vi "Get cyclic instructions.vi"(8 "error in (no error)":errorcluster, 10 "cyclic parameter":string, 11 "Motor in":refnum<class "Motor.lvclass">) -> (0 "error out":errorcluster, 1 "start":bool, 2 "cyclic instructions":string[](array[string]), 3 "Motor out":refnum<class "Motor.lvclass">)   [LabVIEW 2018, in "Motor.lvclass"]
uses:
  Motor.lvclass
  Motor.lvclass/Motor.ctl
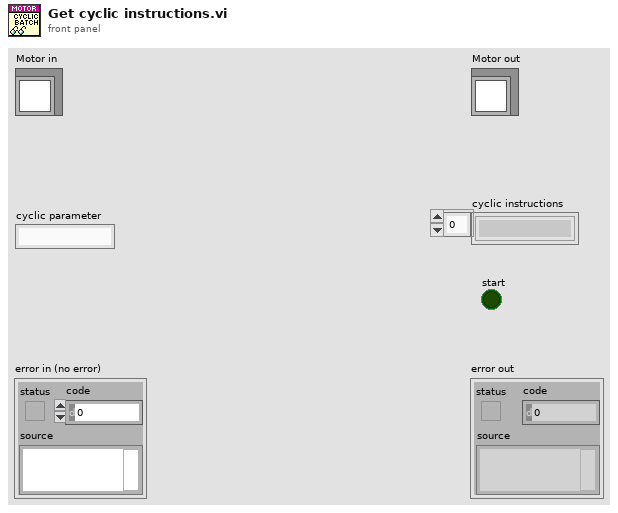
[diagram p1: front panel]
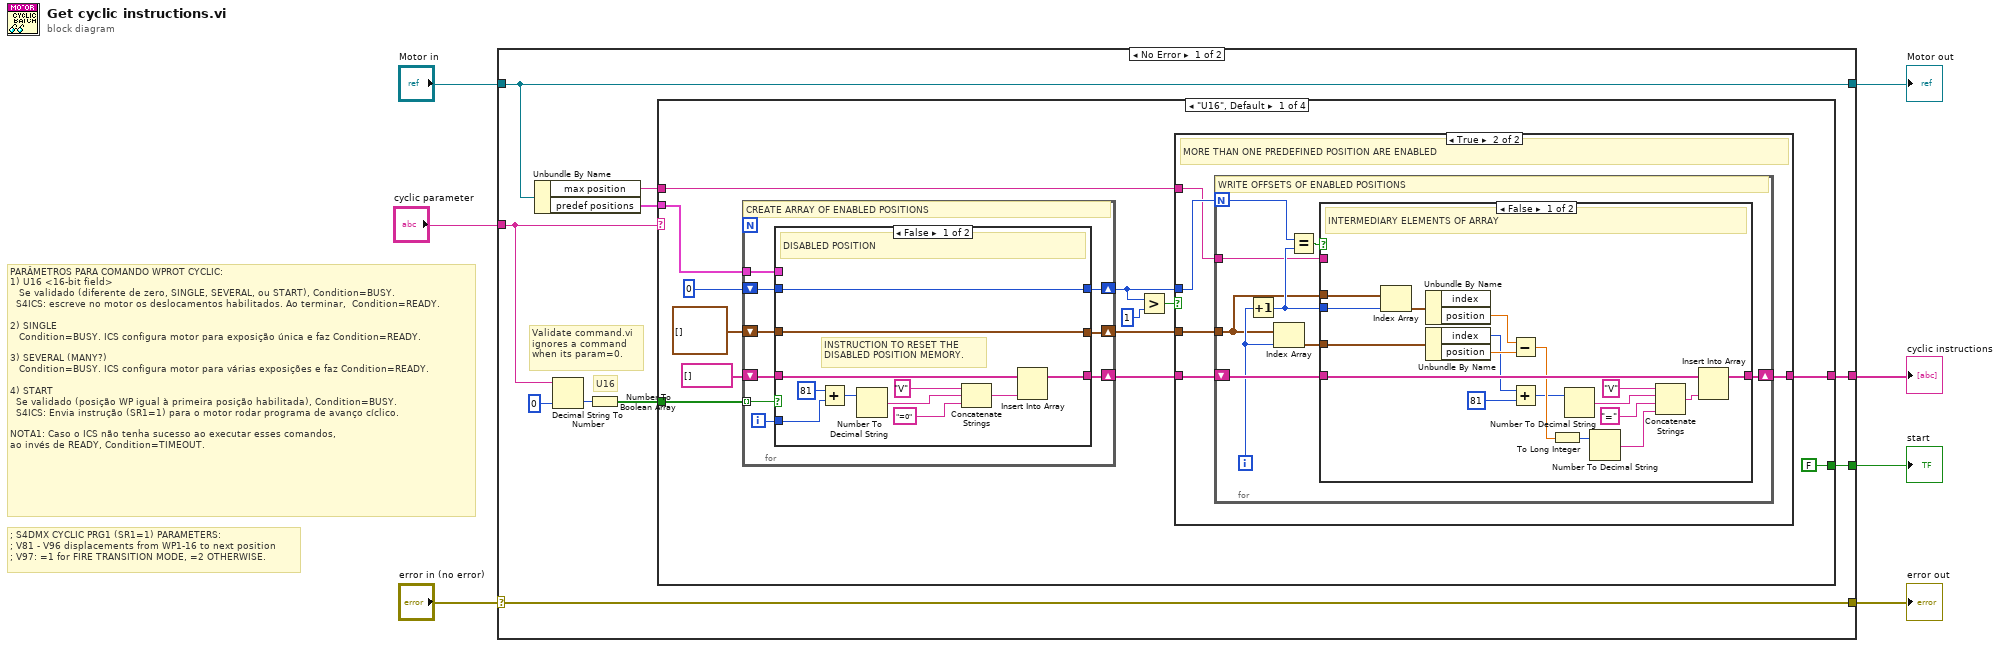
[diagram p0: block diagram]
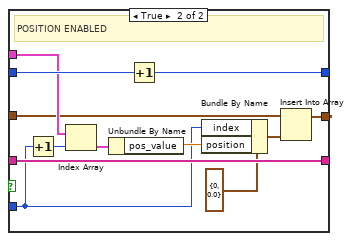
[diagram p2: hidden frame]
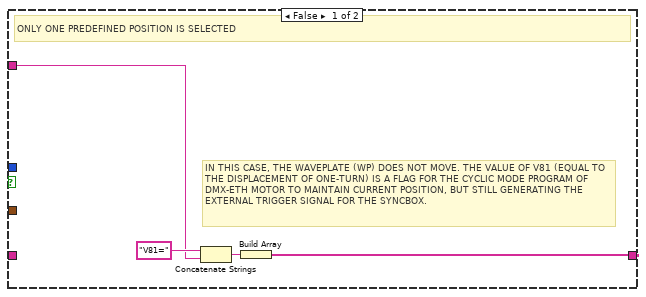
[diagram p3: hidden frame]
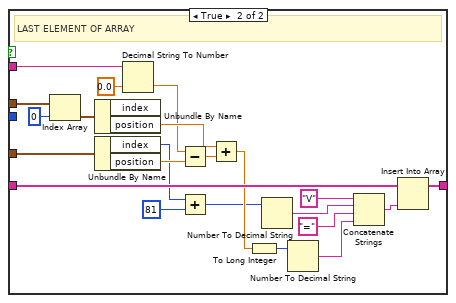
[diagram p4: hidden frame]
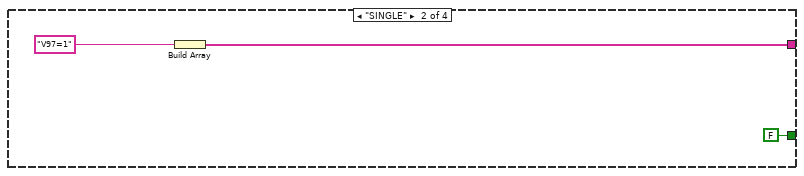
[diagram p5: hidden frame]
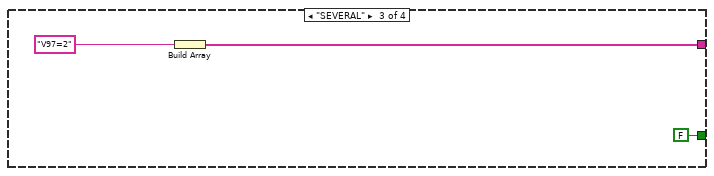
[diagram p6: hidden frame]
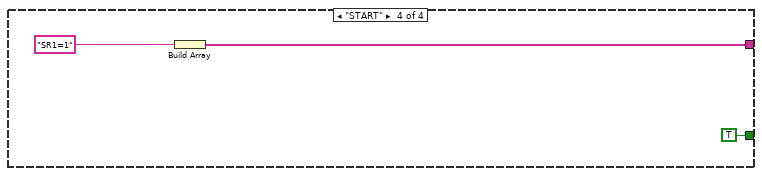
[diagram p7: hidden frame]
diagram:
  # "; S4DMX CYCLIC PRG1 (SR1=1) PARAMETERS:\n; V81 - V96 displacements from WP1-16 to next position\n; V97: =1 for FIRE TRANSITION MODE, =2 OTHERWISE."
  # "PARÂMETROS PARA COMANDO WPROT CYCLIC:\n1) U16 <16-bit field>\n   Se validado (diferente de zero, SINGLE, SEVERAL, ou START), Condition=BUSY.\n  S4ICS: escreve no motor os deslocamentos habilitados. Ao terminar,  Condition=READY.\n\n2) SINGLE\n   Condition=BUSY. ICS configura motor para exposição única e faz Condition=READY.\n\n3) SEVERAL (MANY?)\n   Condition=BUSY. ICS configura motor para várias exposições e faz Condition=READY.\n\n4) START\n  Se validado (posição WP igual à primeira posição habilitada), Condition=BUSY.\n  S4ICS: Envia instrução (SR1=1) para o motor rodar programa de avanço cíclico.\n\nNOTA1: Caso o ICS não tenha sucesso ao executar esses comandos, \nao invés de READY, Condition=TIMEOUT."
  n1 = case shown="No Error" "error in (no error)" {
    selector: "error in (no error)" -> [w17 w130]
    tunnel: [w17 w130] -> w6
    tunnel: [w16 w131] -> w4
    tunnel: "Motor in" -> [w16 w131]
    tunnel: "cyclic parameter" -> [w13 _]
    tunnel: [w9 _] -> w2
    tunnel: [w8 _] -> w1
    frame No Error {
      # "Validate command.vi\nignores a command\nwhen its param=0."
      # "U16"
      n2 = Unbundle By Name(w16) -> ("max position"=w14:string, "predef positions"=w15:cluster{"pos_name":string, "pos_value":dbl}[])
      n3 = Decimal String To Number(string=w13, default (0L)=u16 0) -> (number=w12:u16)  [unwired: 1 in, 1 out]
      n4 = Number To Boolean Array(number=w12) -> (Boolean array=w10:bool[])
      n5 = case shown="\"U16\", Default" w13 {
        tunnel: w15 -> [w26 _ _ _]
        tunnel: w14 -> [w20 _ _ _]
        tunnel: w10 -> [w28 _ _ _]
        tunnel: [w19 w122 w125 w128] -> w9
        tunnel: [FALSE FALSE FALSE TRUE] -> w8
        frame "U16", Default {
          n6 = for {
            tunnel: w28 -> [w37] mode=indexing
            shift-right: [w39] -> w21
            shift-left: u16 0 -> [w38]
            shift-right: [w35] -> w22
            shift-left: string[] [] ("appended array") -> [w36]
            tunnel: w26 -> [w33]
            shift-right: [w31] -> w23
            shift-left: cluster{"index":u16, "position":dbl}[] [] ("enabled array") -> [w32]
            i -> [w34]
            # "CREATE ARRAY OF ENABLED POSITIONS"
            n7 = case shown="False" w37 {
              tunnel: [w50 w62] -> w39
              tunnel: w38 -> [w50 w61]
              tunnel: w36 -> [w43 w60]
              tunnel: [w42 w60] -> w35
              tunnel: w34 -> [w44 w51]
              tunnel: w33 -> [_ w59]
              tunnel: w32 -> [w40 w56]
              tunnel: [w40 w57] -> w31
              frame False {
                # "INSTRUCTION TO RESET THE \nDISABLED POSITION MEMORY."
                # "DISABLED POSITION"
                n8 = Add(x=81, y=w44) -> (x+y=w49:i32)
                n9 = Number To Decimal String(number=w49) -> (decimal integer string=w48:string)  [unwired: 1 in]
                n10 = Concatenate Strings("V", w48, "=0") -> (w41:string)
                n11 = Insert Into Array(array=w43, new element=w41) -> (w42:string[])  [unwired: 1 in]
              }
              frame True {
                # "POSITION ENABLED"
                n12 = Increment(x=w51) -> (x+1=w53:i32)
                n13 = Index Array(array=w59, index=w53) -> (element=w58:cluster{"pos_name":string, "pos_value":dbl})
                n14 = Unbundle By Name(w58) -> ("pos_value"=w54:dbl)
                n15 = Increment(x=w61) -> (x+1=w62:u16)
                n16 = Bundle By Name(cluster=cluster{"index":u16, "position":dbl} {"index"=0, "position"=0.0} ("element"), "index"=w51, "position"=w54) -> (w52:cluster{"index":u16, "position":dbl})
                n17 = Insert Into Array(array=w56, new element=w52) -> (w57:cluster{"index":u16, "position":dbl}[])  [unwired: 1 in]
              }
            }
          }
          n18 = Greater?(x=w21, y=u16 1) -> (0:w30:bool)
          n19 = case shown="True" w30 {
            tunnel: w20 -> [w64 w68]
            tunnel: w23 -> [_ w70]
            tunnel: w22 -> [_ w71]
            tunnel: w21 -> [_ w69]
            tunnel: [w63 w67] -> w19
            frame False {
              # "IN THIS CASE, THE WAVEPLATE (WP) DOES NOT MOVE. THE VALUE OF V81 (EQUAL TO THE DISPLACEMENT OF ONE-TURN) IS A FLAG FOR THE CYCLIC MODE PROGRAM OF DMX-ETH MOTOR TO MAINTAIN CURRENT POSITION, BUT STILL GENERATING THE EXTERNAL TRIGGER SIGNAL FOR THE SYNCBOX."
              # "ONLY ONE PREDEFINED POSITION IS SELECTED"
              n20 = Concatenate Strings("V81=", w64) -> (w66:string)
              n21 = Build Array(w66) -> (w63:string[])
            }
            frame True {
              # "MORE THAN ONE PREDEFINED POSITION ARE ENABLED"
              n22 = for {
                N: w69 -> [w76]
                tunnel: w70 -> [w74]
                shift-right: [w77] -> w67
                shift-left: w71 -> [w79]
                tunnel: w68 -> [w72]
                i -> [w78]
                # "WRITE OFFSETS OF ENABLED POSITIONS"
                n23 = Increment(x=w78) -> (x+1=w75:i32)
                n24 = Index Array(array=w74, index=w78) -> (element=w80:cluster{"index":u16, "position":dbl})
                n25 = Equal?(x=w76, y=w75) -> (x = y?=w73:bool)
                n26 = case shown="False" w73 {
                  tunnel: w80 -> [w98 w120]
                  tunnel: w79 -> [w93 w115]
                  tunnel: [w88 w111] -> w77
                  tunnel: w75 -> [w86 _]
                  tunnel: w74 -> [w85 w110]
                  tunnel: w72 -> [_ w100]
                  frame False {
                    # "INTERMEDIARY ELEMENTS OF ARRAY"
                    n27 = Index Array(array=w85, index=w86) -> (element=w84:cluster{"index":u16, "position":dbl})
                    n28 = Unbundle By Name(w84) -> ("position"=w87:dbl)  [unwired: 1 out]
                    n29 = Unbundle By Name(w98) -> ("index"=w83:u16, "position"=w97:dbl)
                    n30 = Subtract(x=w87, y=w97) -> (x-y=w90:dbl)
                    n31 = Add(x=w83, y=81 ("x")) -> (x+y=w81:i32)
                    n32 = To Long Integer(number=w90) -> (32bit integer=w92:i32)
                    n33 = Number To Decimal String(number=w81) -> (decimal integer string=w94:string)  [unwired: 1 in]
                    n34 = Number To Decimal String(number=w92) -> (decimal integer string=w91:string)  [unwired: 1 in]
                    n35 = Concatenate Strings("V", w94, "=", w91) -> (w89:string)
                    n36 = Insert Into Array(array=w93, new element=w89) -> (w88:string[])  [unwired: 1 in]
                  }
                  frame True {
                    # "LAST ELEMENT OF ARRAY"
                    n37 = Index Array(array=w110, index=0) -> (element=w109:cluster{"index":u16, "position":dbl})
                    n38 = Unbundle By Name(w109) -> ("position"=w106:dbl)  [unwired: 1 out]
                    n39 = Unbundle By Name(w120) -> ("index"=w103:u16, "position"=w119:dbl)
                    n40 = Decimal String To Number(string=w100, default (0L)=0.0) -> (number=w99:dbl)  [unwired: 1 in, 1 out]
                    n41 = Subtract(x=w99, y=w119) -> (x-y=w107:dbl)
                    n42 = Add(x=w103, y=u16 81) -> (x+y=w104:u16)
                    n43 = Add(x=w106, y=w107) -> (x+y=w105:dbl)
                    n44 = To Long Integer(number=w105) -> (32bit integer=w114:i32)
                    n45 = Number To Decimal String(number=w104) -> (decimal integer string=w116:string)  [unwired: 1 in]
                    n46 = Number To Decimal String(number=w114) -> (decimal integer string=w113:string)  [unwired: 1 in]
                    n47 = Concatenate Strings("V", w116, "=", w113) -> (w112:string)
                    n48 = Insert Into Array(array=w115, new element=w112) -> (w111:string[])  [unwired: 1 in]
                  }
                }
              }
            }
          }
        }
        frame "SINGLE" {
          n49 = Build Array("V97=1" ("string")) -> (w122:string[])
        }
        frame "SEVERAL" {
          n50 = Build Array("V97=2" ("string")) -> (w125:string[])
        }
        frame "START" {
          n51 = Build Array("SR1=1" ("string")) -> (w128:string[])
        }
      }
    }
    frame Error {
    }
  }
  "error out" <- w6
  "Motor out" <- w4
  "cyclic instructions" <- w2
  "start" <- w1
